vi "Verify threshold value by repeated iteration.vi"(4 "Cluster":T1={"Delta Matrix "=[[-1.0, 0.0, 0.0, 0.0, 0.0, 0.0, 0.0, 0.0, 0.0], [0.0, -1.0, 0.0, 0.0, 0.0, 0.0, 0.0, 0.0, 0.0], [0.0, 0.0, 0.0, 0.0, 0.0, 0.0, 0.0, 0.0, 0.0], [0.0, 0.0, 0.0, 0.0, 0.0, 0.0, 0.0, 0.0, 0.0], [10.0, 0.0, 0.0, 0.0, 0.0, 0.0, 0.0, 0.0, 0.0], [10.0, 0.0, 0.0, 0.0, 0.0, 0.0, 0.0, 0.0, 0.0], [0.0, 10.0, 0.0, 0.0, 0.0, 0.0, 0.0, 0.0, 0.0]], "Idx of Mod in Sp IDs "=[2, 8], "idx of OP "=0, "Init Sp State "=[], "Equations "=["kd*CI", "kd*GFP", "kd*LacI", "kd*TetR", "(ko__P1*ng__P1*Ko__P1*RNAP)/(1+Ko__P1*RNAP+(Kr__LacI_P1*LacI)^nc__LacI_P1)", "(ko__P2*ng__P2*Ko__P2*RNAP)/(1+Ko__P2*RNAP+(Kr__TetR_P2*TetR)^nc__TetR_P2)", "(ko__Promoter_GFP*ng__Promoter_GFP*Ko__Promoter_GFP*RNAP)/(1+Ko__Promoter_GFP*RNAP+(Kr__CI_Promoter_GFP*CI)^nc__CI_Promoter_GFP)"], "All Param Names "=[], "All Param Values "=[], "Sp Ids "=["CI", "GFP", "LacI", "P1", "P2", "P3", "P3_mRNA", "Promoter_GFP", "TetR"], "Start at "=0.0, "Pos Thresh "=10.0, "Runs "=0.0, "Init OP Conc "=0.0, "Comb "="", "Verification RT "=0.0, "CompID"=[], "CompSize"=[], "ModTimeSym"="", "Settling Time"=10}) -> (0 "T-Delay-SD":dbl format="%0.2f", 1 "OP Consistency":dbl, 2 "T-delay.av":i32)   [LabVIEW 2014]
doc: "This VI verifies the expected threshold value by iterating the model for the specified number of times. It also estimates the propogation delay (or input-output time delay). \n\nDesigned by HB\nhaba@dtu.dk"
uses:
  <vilib>/Analysis/Matrix/Datatypes/RealMatrix.ctl
  VerifyThreshInpCtrl.ctl
  ValSubsCtrl.ctl
  Trigger Status Bar.vi
  <vilib>/Analysis/Matrix/Numeric/Conversions/Matrix To Array - RM.vi
  <vilib>/gmath/NI_Gmath.lvlib
  <vilib>/Analysis/Matrix/NI_Matrix.lvlib
  <vilib>/Analysis/NI_AALBase.lvlib
panel:
  out "TIME IN MS":i32
  out "Time offset":i32=10
  out "T-Delay 2":dbl[](array[numeric])
  out "Zeros":dbl
  out "TD-Idxs":i32[](array[numeric])
  out "T-Delay":dbl[](array[numeric])
  out "Th-Var.av":dbl format="%0.2f"
  out "Th-SD.av":dbl format="%0.2f"
  out "Var":dbl[](array[numeric])
  out "SD":dbl[](array[numeric])
  out "ModTimeSym":string
  out "CompSize":string[](array[string])
  out "CompID":string[](array[string])
  out "Verification RT":dbl
  out "No. of inputs":i32
  out "Comb":string
  out "Init OP Conc":dbl
  out "Var Cnt":i32
  out "T-Delay Idx":i32
  out "Q":dbl
  out "O/p int Matrix":dbl[][](array[numeric]) format="%0.3f"
  out "Time int Matrix":dbl[][](array[numeric]) format="%0.3f"
  out "OP int data":dbl[](array[numeric])
  out "idx":i32
  out "T-Interval":dbl[](array[numeric])
  out "Q-Check":i32
  out "Time Matrix":dbl[][](array[numeric]) format="%0.3f"
  out "Time array":dbl[](array[numeric])
  in  "Print Interval":dbl=10.0
  out "OP Av":dbl[](array[numeric])
  out "Run":i32
  out "Init Sp State":i32[](array[numeric])
  out "Runs":dbl
  out "Log Data Nxt":dbl[](array[numeric])
  out "Log Data matrix 2":dbl[][](array[numeric]) format="%0.3f"
  out "OP Data":dbl[](array[numeric])
  out "O/p Matrix":dbl[][](array[numeric]) format="%0.3f"
  out "Pos Thresh":dbl=10.0
  out "Start at":dbl
  out "idx of OP":i32
  out "Mod data":dbl[](array[numeric])
  out "Sp Ids":string[](array[string])=["CI", "GFP", "LacI", "P1", "P2", "P3", "P3_mRNA", "Promoter_GFP", "TetR"]
  out "All Param Names":string[](array[string])
  out "All Param Values":string[](array[string])
  out "Nxt Sp State (N)":dbl[](array[numeric])
  out "Nxt Sp State (S)":string[](array[string])
  out "Idx of Mod in Sp IDs":i32[](array[numeric])=[2, 8]
  out "Nxt T":dbl
  out "Sum of Propensities for U":dbl
  out "Reac to execute":dbl[](array[numeric])
  out "Sum>a0*r2":bool
  out "Delta Matrix":T2=[[-1.0, 0.0, 0.0, 0.0, 0.0, 0.0, 0.0, 0.0, 0.0], [0.0, -1.0, 0.0, 0.0, 0.0, 0.0, 0.0, 0.0, 0.0], [0.0, 0.0, 0.0, 0.0, 0.0, 0.0, 0.0, 0.0, 0.0], [0.0, 0.0, 0.0, 0.0, 0.0, 0.0, 0.0, 0.0, 0.0], [10.0, 0.0, 0.0, 0.0, 0.0, 0.0, 0.0, 0.0, 0.0], [10.0, 0.0, 0.0, 0.0, 0.0, 0.0, 0.0, 0.0, 0.0], [0.0, 10.0, 0.0, 0.0, 0.0, 0.0, 0.0, 0.0, 0.0]]
  out "Reac IDx":i32
  out "a0*r2":dbl
  out "r1":dbl
  out "a0":dbl
  out "Propensities":dbl[](array[numeric])
  out "L_cnt":i32
  out "T":dbl[](array[numeric])
  out "tau":dbl
  out "r2":dbl
  out "Equations":string[](array[string])=["kd*CI", "kd*GFP", "kd*LacI", "kd*TetR", "(ko__P1*ng__P1*Ko__P1*RNAP)/(1+Ko__P1*RNAP+(Kr__LacI_P1*LacI)^nc__LacI_P1)", "(ko__P2*ng__P2*Ko__P2*RNAP)/(1+Ko__P2*RNAP+(Kr__TetR_P2*TetR)^nc__TetR_P2)", "(ko__Promoter_GFP*ng__Promoter_GFP*Ko__Promoter_GFP*RNAP)/(1+Ko__Promoter_GFP*RNAP+(Kr__CI_Promoter_GFP*CI)^nc__CI_Promoter_GFP)"]
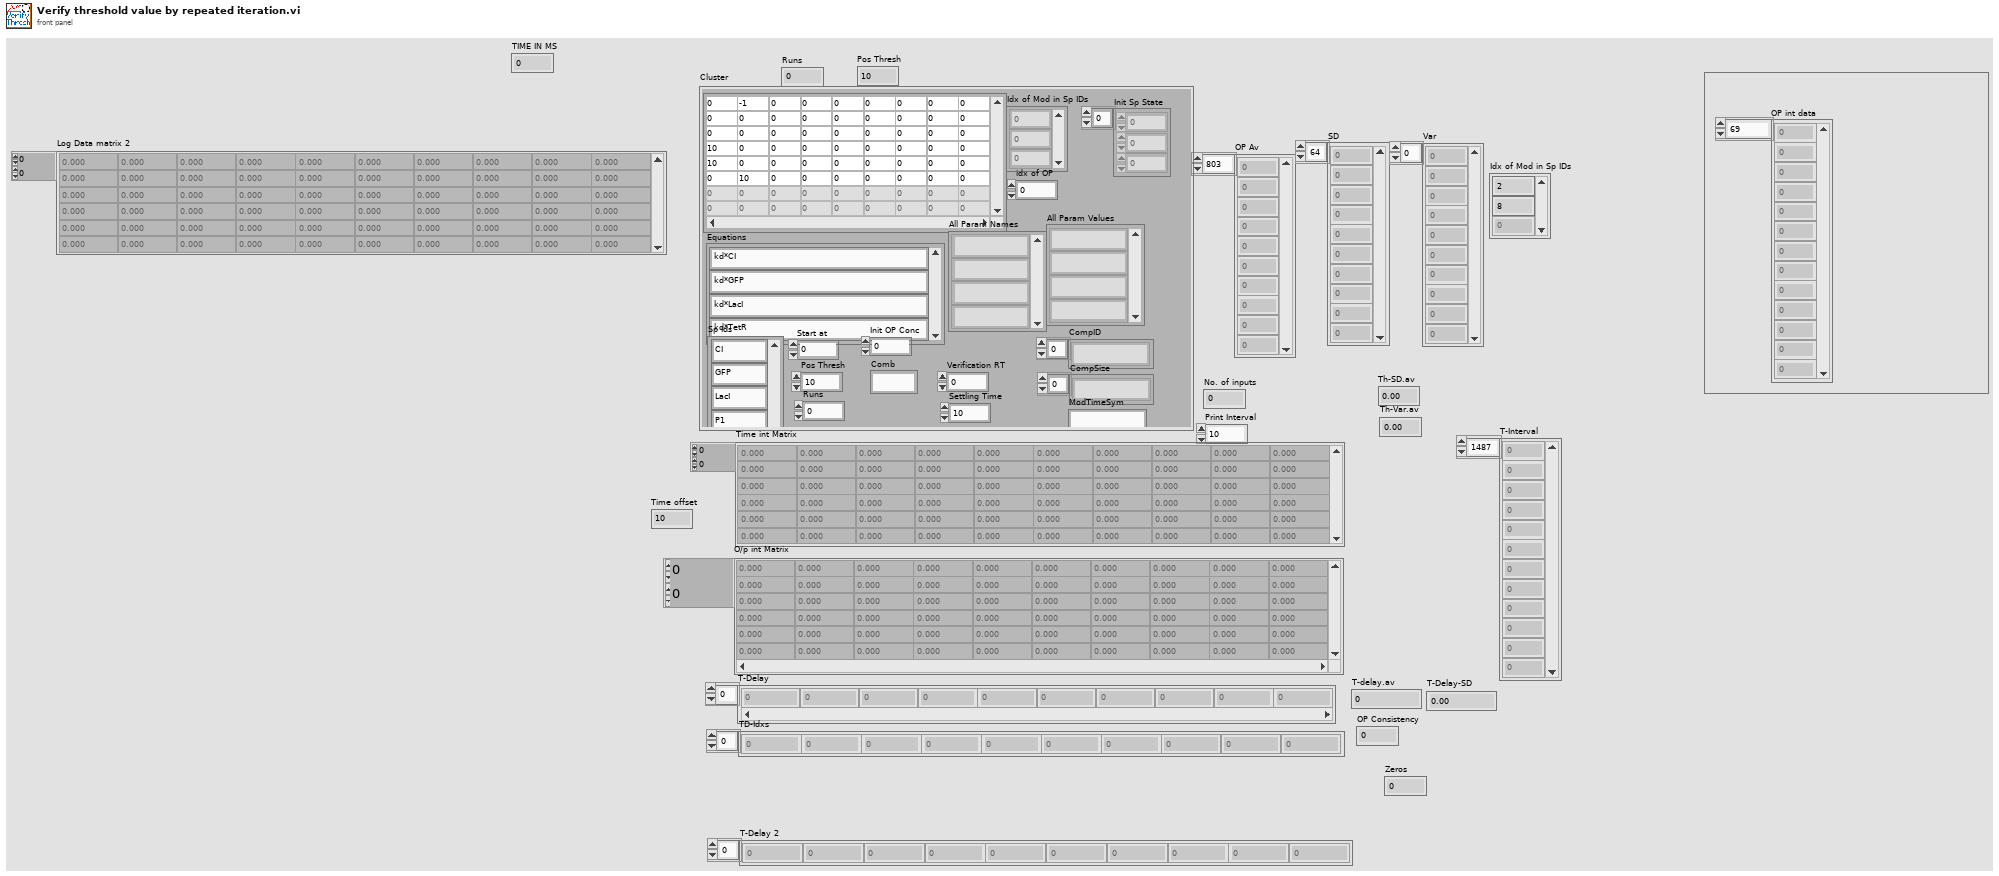
[diagram p1: front panel]
types:
  T1 = typedef "VerifyThreshInpCtrl.ctl" = cluster{"Delta Matrix ":T2, "Idx of Mod in Sp IDs ":i32[], "idx of OP ":i32, "Init Sp State ":i32[], "Equations ":string[], "All Param Names ":string[], "All Param Values ":string[], "Sp Ids ":string[], "Start at ":dbl, "Pos Thresh ":dbl, "Runs ":dbl, "Init OP Conc ":dbl, "Comb ":string, "Verification RT ":dbl, "CompID":string[], "CompSize":string[], "ModTimeSym":string, "Settling Time":i32}
  T2 = typedef "NI_Matrix.lvlib/RealMatrix.ctl" = dbl[][]
  T3 = typedef "ValSubsCtrl.ctl" = cluster{"All Param Names":string[], "All Param Values":string[], "Sp IDs":string[], "Sp States":string[], "Input Equations":string[], "CompID":string[], "CompSize":string[], "T-Sym":string, "T":dbl}
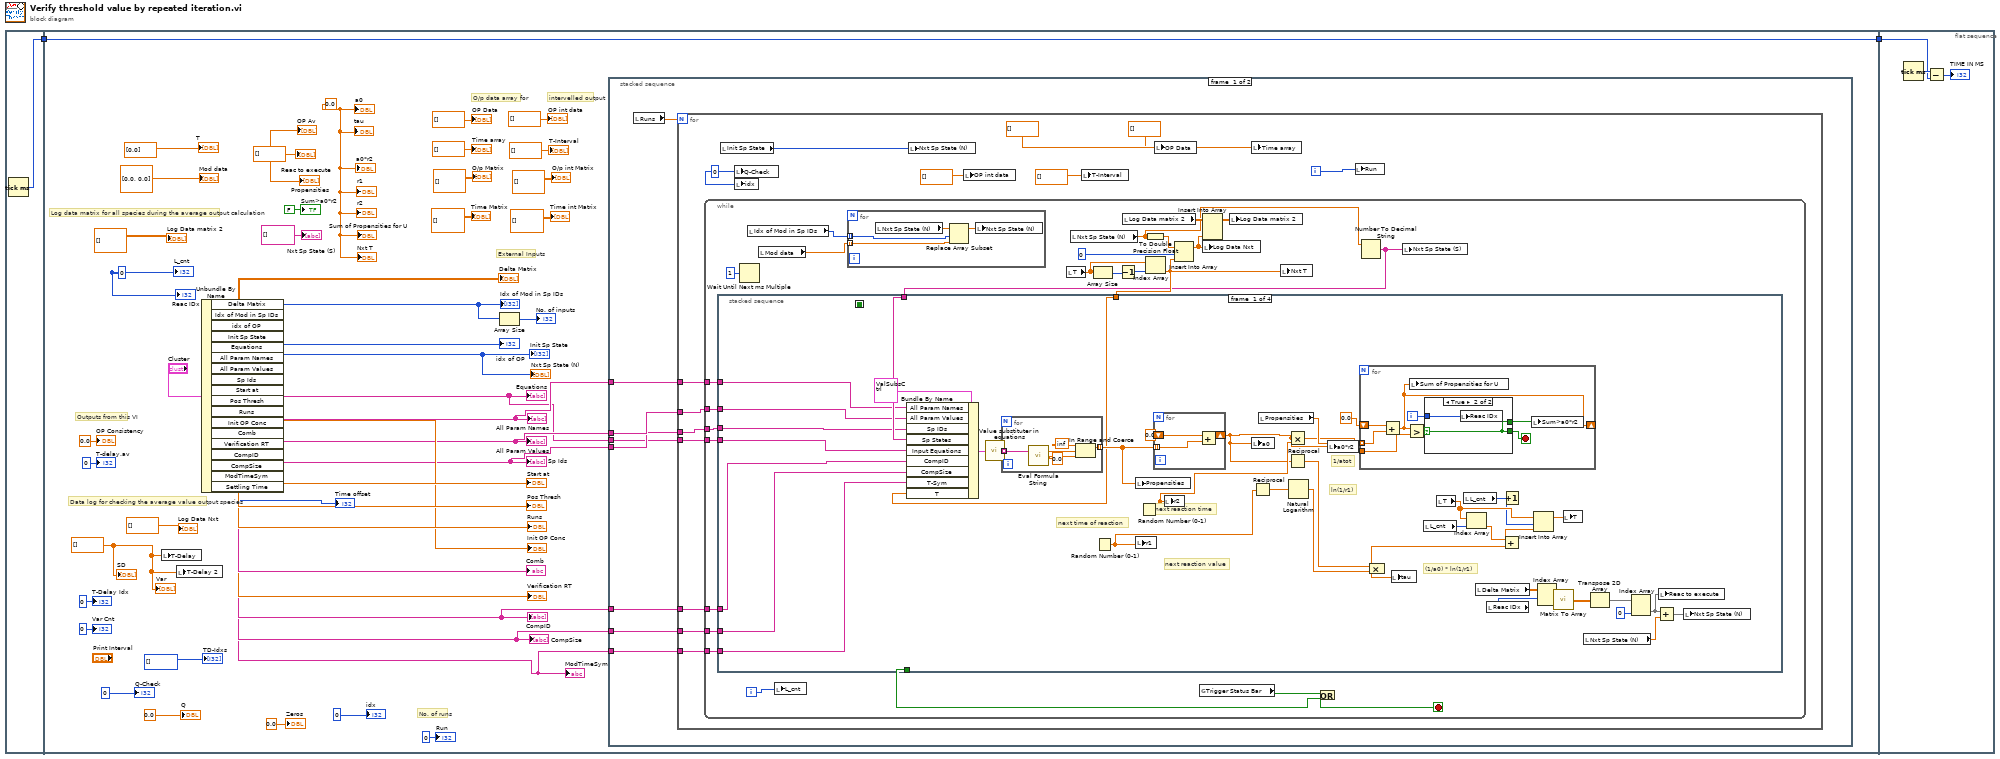
[diagram p0: block diagram]
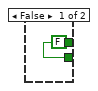
[diagram p2: hidden frame]
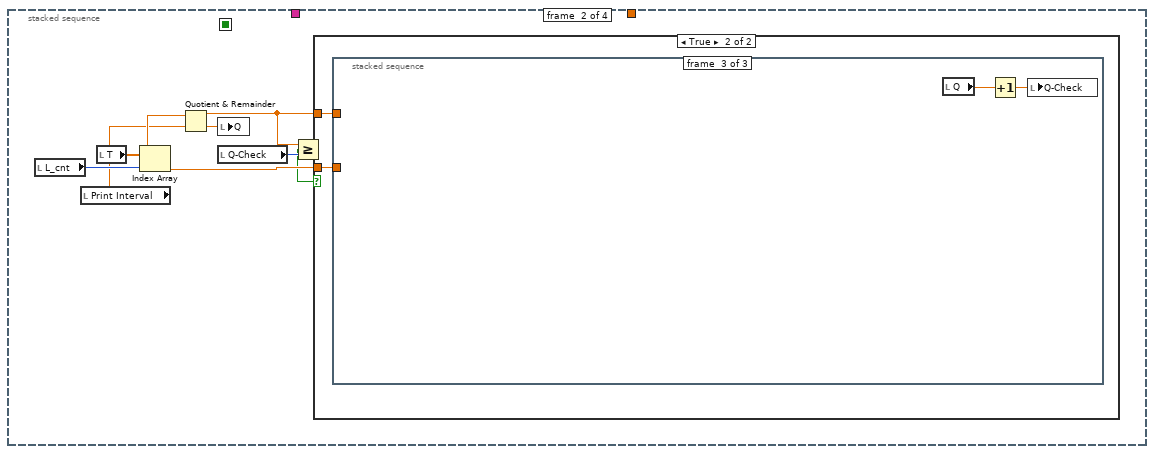
[diagram p3: hidden frame]
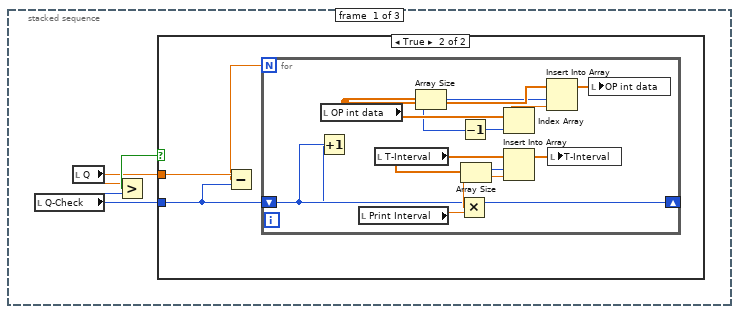
[diagram p5: hidden frame]
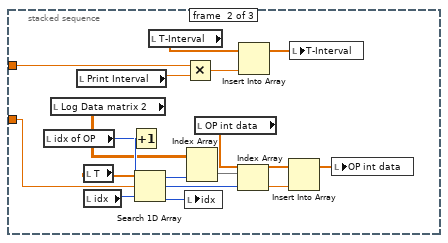
[diagram p7: hidden frame]
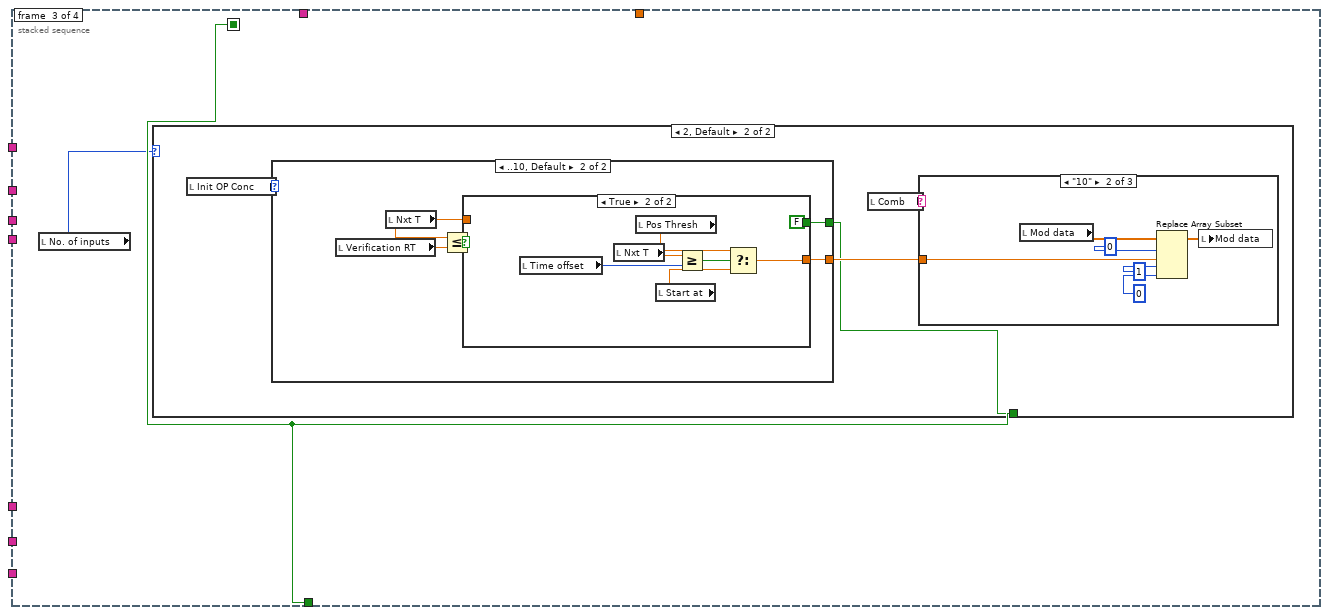
[diagram p8: hidden frame]
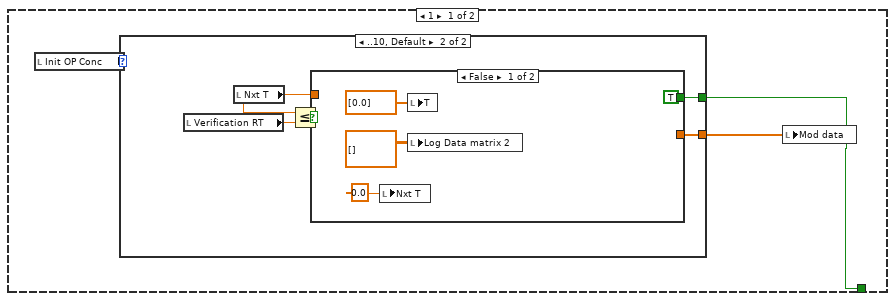
[diagram p9: hidden frame]
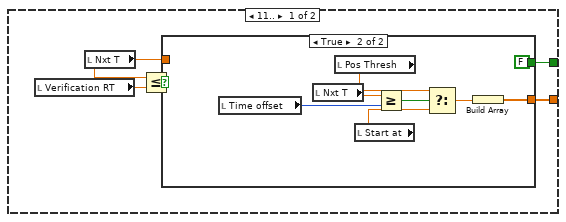
[diagram p10: hidden frame]
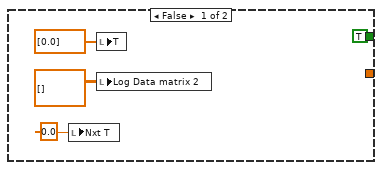
[diagram p11: hidden frame]
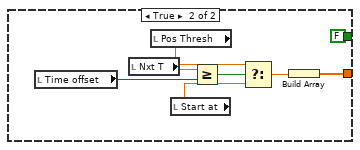
[diagram p12: hidden frame]
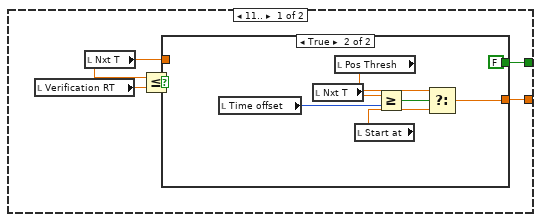
[diagram p13: hidden frame]
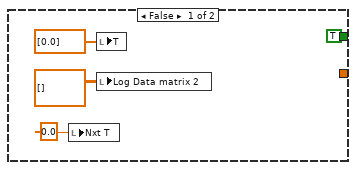
[diagram p14: hidden frame]
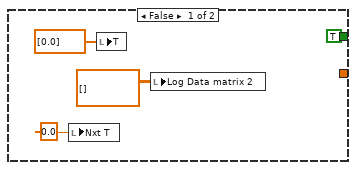
[diagram p15: hidden frame]
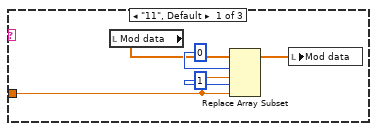
[diagram p16: hidden frame]
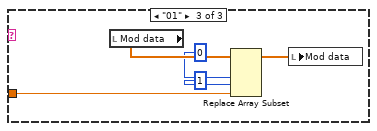
[diagram p17: hidden frame]
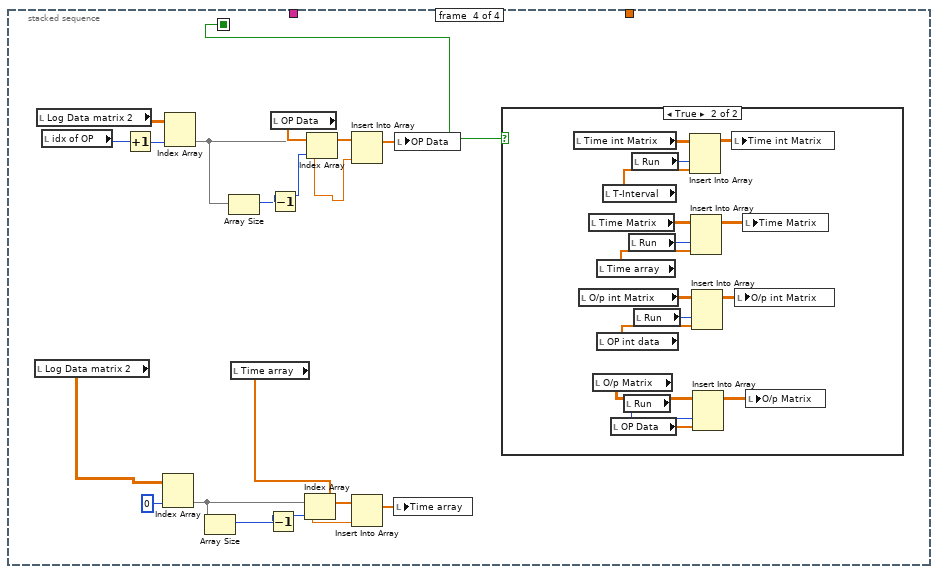
[diagram p18: hidden frame]
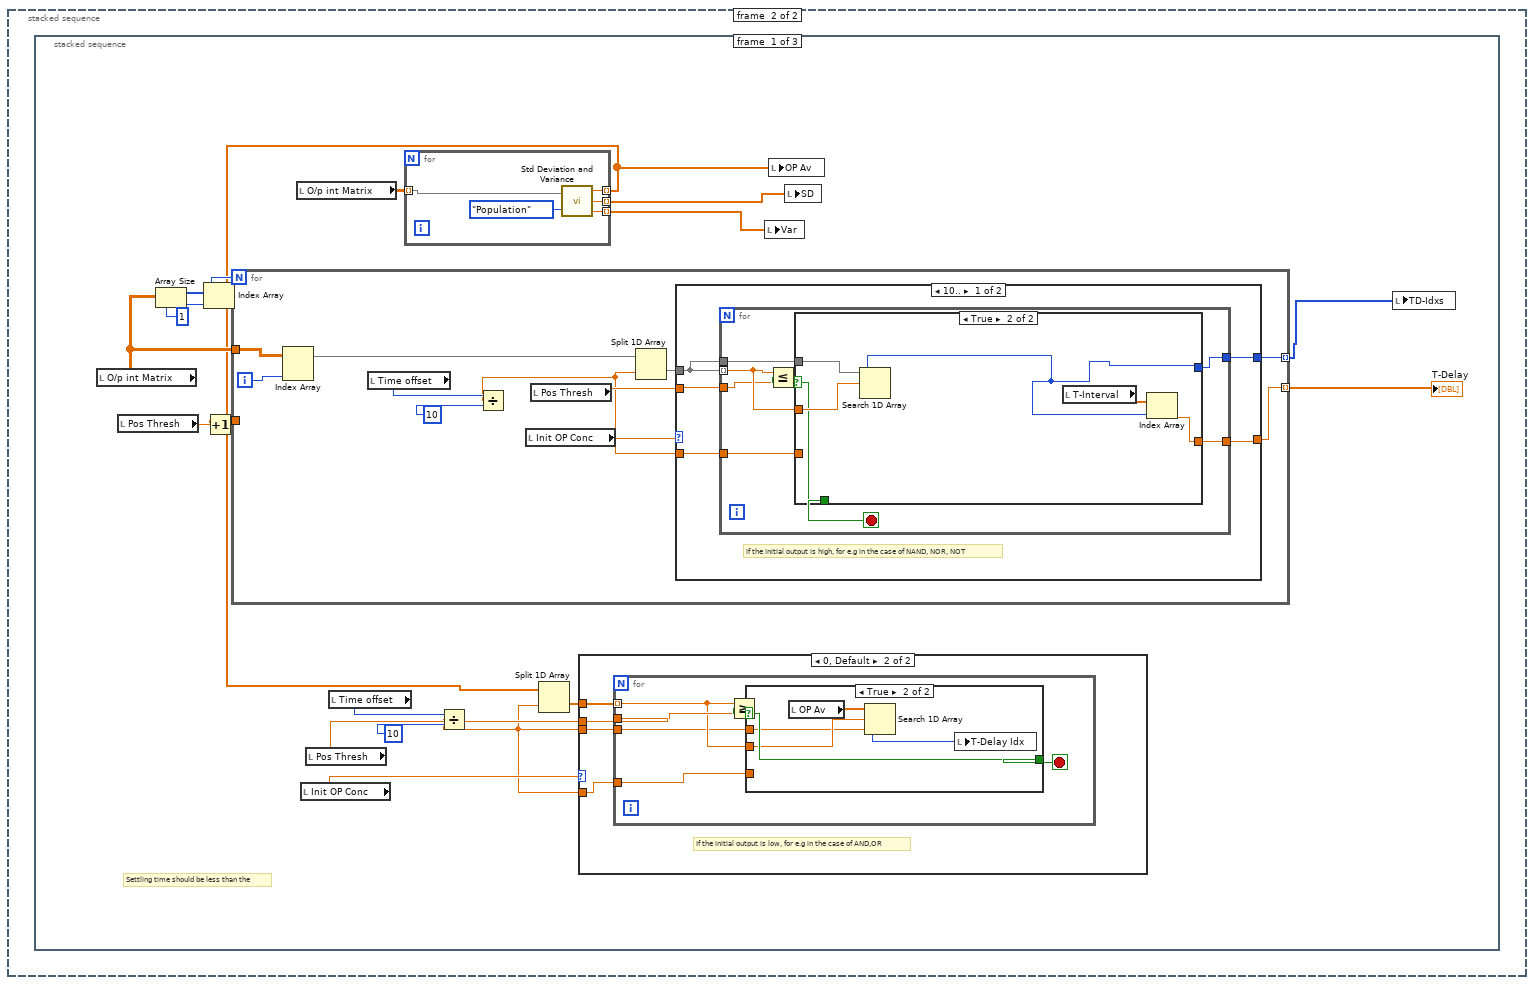
[diagram p20: hidden frame]
diagram:
  n1 = flat-sequence {
    tunnel: [w3] -> w1
    tunnel: [w11] -> w2
    tunnel: w1 -> [w11]
    tunnel: w2 -> [w514]
    frame #0 {
      n2 = Tick Count (ms)() -> (millisecond timer value=w3:u32)
    }
    frame #1 {
      w13 = dbl[] [] ("Var")
      w43 = 0 ("L_cnt")
      w41 = dbl[] [] ("Reac to execute")
      w47 = 0.0 ("a0")
      # "Outputs from this VI"
      # "intervelled output"
      # "No. of runs"
      # "External Inputs"
      # "O/p data array for"
      # "Log data matrix for all species during the average output calculation"
      # "Data log for checking the average value output species"
      n3 = local write "T-Delay"(w13) -> ()
      n4 = local write "T-Delay 2"(w13) -> ()
      n5 = Unbundle By Name("Cluster") -> ("Delta Matrix"=→"Delta Matrix":T2, "Idx of Mod in Sp IDs"=w24:i32[], "idx of OP"=→"idx of OP":i32, "Init Sp State"=→"Nxt Sp State (N)" →"Init Sp State":i32[], "Equations"=w7:string[], "All Param Names"=w10:string[], "All Param Values"=w9:string[], "Sp Ids"=w8:string[], "Start at"=→"Start at":dbl, "Pos Thresh"=→"Pos Thresh":dbl, "Runs"=→"Runs":dbl, "Init OP Conc"=→"Init OP Conc":dbl, "Comb"=→"Comb":string, "Verification RT"=→"Verification RT":dbl, "CompID"=w6:string[], "CompSize"=w5:string[], "ModTimeSym"=w4:string, "Settling Time"=→"Time offset":i32)
      "Equations" <- w7
      "Idx of Mod in Sp IDs" <- w24
      "All Param Values" <- w9
      "All Param Names" <- w10
      "Sp Ids" <- w8
      "CompID" <- w6
      "CompSize" <- w5
      "ModTimeSym" <- w4
      n6 = Array Size(array=w24) -> (size(s)=→"No. of inputs":i32)
      n7 = stacked-sequence {
        tunnel: w10 -> [w59 _]
        tunnel: w9 -> [w58 _]
        tunnel: w8 -> [w57 _]
        tunnel: w7 -> [w56 _]
        tunnel: w6 -> [w55 _]
        tunnel: w5 -> [w54 _]
        tunnel: w4 -> [w53 _]
        frame #0 {
          n8 = local read "Runs"() -> (w60:dbl)
          n9 = for {
            N: w60 -> [_]
            tunnel: w59 -> [w67]
            tunnel: w58 -> [w66]
            tunnel: w57 -> [w65]
            tunnel: w56 -> [w64]
            tunnel: w55 -> [w63]
            tunnel: w54 -> [w62]
            tunnel: w53 -> [w61]
            i -> [w73]
            w68 = 0 ("Q-Check")
            n10 = while {
              tunnel: w67 -> [w81]
              tunnel: w66 -> [w80]
              tunnel: w65 -> [w79]
              tunnel: w64 -> [w78]
              tunnel: w63 -> [w77]
              tunnel: w62 -> [w76]
              tunnel: w61 -> [w75]
              i -> [w99]
              stop <- w95 stop-if-true
              n11 = Wait Until Next ms Multiple(millisecond multiple=u32 1) -> ()  [unwired: 1 out]
              n12 = local read "Idx of Mod in Sp IDs"() -> (w93:i32[])
              n13 = local read "Mod data"() -> (w94:dbl[])
              n14 = local write "L_cnt"(w99) -> ()
              n15 = for {
                tunnel: w93 -> [w102] mode=indexing
                tunnel: w94 -> [w100] mode=indexing
                n16 = local read "Nxt Sp State (N)"() -> (w103:dbl[])
                n17 = Replace Array Subset(array=w103, new element=w100, index=w102) -> (w101:dbl[])
                n18 = local write "Nxt Sp State (N)"(w101) -> ()
              }
              n19 = local read "T"() -> (w92:dbl[])
              n20 = local read "Nxt Sp State (N)"() -> (w84:dbl[])
              n21 = Array Size(array=w92) -> (size(s)=w91:i32)
              n22 = Decrement(x=w91) -> (x-1=w90:i32)
              n23 = local read "Log Data matrix 2"() -> (w87:dbl[][])
              n24 = To Double Precision Float(number=w84) -> (double precision float=w88:dbl[])
              n25 = Index Array(array=w92, index=w90) -> (element=w83:dbl)
              n26 = Insert Into Array(array=w88, index=0, new element=w83) -> (w85:dbl[])
              n27 = global read "Trigger Status Bar.vi" "Trigger Status Bar"() -> (w96:bool)
              n28 = Insert Into Array(array=w87, new element=w85) -> (w86:dbl[][])  [unwired: 2 in]
              n29 = local write "Log Data Nxt"(w85) -> ()
              n30 = local write "Log Data matrix 2"(w86) -> ()
              n31 = local write "Nxt T"(w83) -> ()
              n32 = Number To Decimal String(number=w84) -> (decimal integer string=w82:string[])  [unwired: 1 in]
              n33 = stacked-sequence {
                seq-local: [_ _ w209 _] -> [_ _ _ w313]
                tunnel: [_ _ w209 _] -> w97
                tunnel: w83 -> [w112 _ _ _]
                tunnel: w82 -> [w111 _ _ _]
                tunnel: w81 -> [w110 _ _ _]
                tunnel: w80 -> [w109 _ _ _]
                tunnel: w79 -> [w108 _ _ _]
                tunnel: w78 -> [w107 _ _ _]
                tunnel: w77 -> [w106 _ _ _]
                tunnel: w76 -> [w105 _ _ _]
                tunnel: w75 -> [w104 _ _ _]
                frame #0 {
                  # "next time of reaction"
                  # "next reaction value"
                  # "(1/a0) * ln(1/r1)"
                  # "1/atot"
                  # "ln(1/r1)"
                  # "next reaction time"
                  n34 = Bundle By Name(cluster=T3 {"All Param Names"=["k1"], "All Param Values"=["1.5"], "Sp IDs"=["S1", "S2", "S3"], "Sp States"=["0.000000", "0.000000", "0.000000"], "Input Equations"=["C*k1*S1", "1.5*exp(time)^(-1)"], "CompID"=["C"], "CompSize"=["3.0"], "T-Sym"="time", "T"=0.0} ("Cluster"), "All Param Names"=w110, "All Param Values"=w109, "Sp IDs"=w108, "Sp States"=w111, "Input Equations"=w107, "CompID"=w106, "CompSize"=w105, "T-Sym"=w104, "T"=w112) -> (w140:T3)
                  n35 = call "Value substituter in equations.vi"("Cluster"=w140) -> ("Output Equations"=w143:string[])
                  n36 = for {
                    tunnel: w143 -> [w162] mode=indexing
                    tunnel: [w158] -> w142 mode=indexing
                    n37 = call <vilib>:"Eval Formula String.vi"("formula"=w162) -> ("y value"=w159:dbl)  [unwired: 1 in, 1 out]
                    n38 = In Range and Coerce(upper limit=inf, x=w159, lower limit=0.0) -> (coerced(x)=w158:dbl)  [unwired: 1 out]
                  }
                  n39 = Random Number (0-1)() -> (number: 0 to 1=w136:dbl)
                  n40 = local write "Propensities"(w142) -> ()
                  n41 = local write "r1"(w136) -> ()
                  n42 = Random Number (0-1)() -> (number: 0 to 1=w137:dbl)
                  n43 = for {
                    tunnel: w142 -> [w157] mode=indexing
                    shift-right: [w156] -> w126
                    shift-left: 0.0 -> [w155]
                    n44 = Add(x=w155, y=w157) -> (x+y=w156:dbl)
                  }
                  n45 = local write "r2"(w137) -> ()
                  n46 = local write "a0"(w126) -> ()
                  n47 = Reciprocal(x=w136) -> (1/x=w127:dbl)
                  n48 = local read "Propensities"() -> (w124:dbl[])
                  n49 = Multiply(x=w126, y=w137) -> (x*y=w123:dbl)
                  n50 = Reciprocal(x=w126) -> (1/x=w128:dbl)
                  n51 = Natural Logarithm(1:w127) -> (0:w129:dbl)
                  n52 = local write "a0*r2"(w123) -> ()
                  n53 = for {
                    tunnel: w124 -> [w148] mode=indexing
                    shift-right: [w147] -> _
                    shift-left: 0.0 -> [w151]
                    tunnel: w123 -> [w144]
                    i -> [w145]
                    stop <- w149 stop-if-true
                    n54 = Add(x=w151, y=w148) -> (x+y=w147:dbl)
                    n55 = Greater?(x=w147, y=w144) -> (0:w150:bool)
                    n56 = local write "Sum of Propensities for U"(w147) -> ()
                    n57 = case shown="True" w150 {
                      selector: w150 -> [_ w154]
                      tunnel: [w152 w154] -> w149
                      tunnel: [w152 w154] -> w146
                      tunnel: w145 -> [_ w153]
                      frame False {
                        w152 = FALSE
                      }
                      frame True {
                        n58 = local write "Reac IDx"(w153) -> ()
                      }
                    }
                    n59 = local write "Sum>a0*r2"(w146) -> ()
                  }
                  n60 = Compound Arithmetic op=MULTIPLY(w128, w129) -> (w122:dbl)
                  n61 = local write "tau"(w122) -> ()
                  n62 = local read "L_cnt"() -> (w132:i32)
                  n63 = local read "T"() -> (w138:dbl[])
                  n64 = local read "L_cnt"() -> (w134:i32)
                  n65 = Index Array(array=w138, index=w132) -> (element=w131:dbl)
                  n66 = local read "Delta Matrix"() -> (w113:T2)
                  n67 = local read "Reac IDx"() -> (w114:i32)
                  n68 = Add(x=w131, y=w122) -> (x+y=w133:dbl)
                  n69 = Increment(x=w134) -> (x+1=w130:i32)
                  n70 = Insert Into Array(array=w138, index=w130, new element=w133) -> (w135:dbl[])
                  n71 = Index Array(array=w113, index (row)=w114) -> (element=w115:T2)  [unwired: 1 in]
                  n72 = call-poly <vilib>:"Matrix To Array.vi"("Real Matrix"=w115) -> ("Real 2D Array"=w116:dbl[][])
                  n73 = local write "T"(w135) -> ()
                  n74 = local read "Nxt Sp State (N)"() -> (w119:dbl[])
                  n75 = Transpose 2D Array(2D array=w116) -> (transposed array=w117:dbl[][])
                  n76 = Index Array(array=w117, index (col)=0 ("disabled index (col)")) -> (element=w121:dbl[])  [unwired: 1 in]
                  n77 = Add(x=w121, y=w119) -> (x+y=w120:dbl[])
                  n78 = local write "Reac to execute"(w121) -> ()
                  n79 = local write "Nxt Sp State (N)"(w120) -> ()
                }
                frame #1 {
                  n80 = local read "L_cnt"() -> (w168:i32)
                  n81 = local read "Print Interval"() -> (w166:dbl)
                  n82 = local read "T"() -> (w167:dbl[])
                  n83 = Index Array(array=w167, index=w168) -> (element=w169:dbl)
                  n84 = Quotient & Remainder(x=w169, y=w166) -> (floor(x/y)=w163:dbl)  [unwired: 1 out]
                  n85 = local write "Q"(w163) -> ()
                  n86 = local read "Q-Check"() -> (w165:i32)
                  n87 = Greater Or Equal?(x=w163, y=w165) -> (x >= y?=w164:bool)
                  n88 = case shown="True" w164 {
                    tunnel: w169 -> [_ w171]
                    tunnel: w163 -> [_ w170]
                    frame False {
                    }
                    frame True {
                      n89 = stacked-sequence {
                        tunnel: w171 -> [_ w204 _]
                        tunnel: w170 -> [_ w190 _]
                        frame #0 {
                          n90 = local read "Q-Check"() -> (w172:i32)
                          n91 = local read "Q"() -> (w173:dbl)
                          n92 = Greater?(x=w173, y=w172) -> (0:w174:bool)
                          n93 = case shown="True" w174 {
                            tunnel: w173 -> [_ w177]
                            tunnel: w172 -> [_ w175]
                            frame False {
                            }
                            frame True {
                              n94 = Subtract(x=w177, y=w175) -> (x-y=w176:dbl)
                              n95 = for {
                                N: w176 -> [_]
                                shift-right: [w184] -> _
                                shift-left: w175 -> [w185]
                                n96 = Increment(x=w185) -> (x+1=w184:i32)
                                n97 = local read "OP int data"() -> (w182:dbl[])
                                n98 = local read "Print Interval"() -> (w189:dbl)
                                n99 = local read "T-Interval"() -> (w186:dbl[])
                                n100 = Array Size(array=w182) -> (size(s)=w178:i32)
                                n101 = Multiply(x=w185, y=w189) -> (x*y=w187:dbl)
                                n102 = Decrement(x=w178) -> (x-1=w181:i32)
                                n103 = Array Size(array=w186) -> (size(s)=w179:i32)
                                n104 = Index Array(array=w182, index=w181) -> (element=w180:dbl)
                                n105 = Insert Into Array(array=w186, index=w179, new element=w187) -> (w188:dbl[])
                                n106 = Insert Into Array(array=w182, index=w178, new element=w180) -> (w183:dbl[])
                                n107 = local write "T-Interval"(w188) -> ()
                                n108 = local write "OP int data"(w183) -> ()
                              }
                            }
                          }
                        }
                        frame #1 {
                          n109 = local read "idx of OP"() -> (w201:i32)
                          n110 = local read "Log Data matrix 2"() -> (w200:dbl[][])
                          n111 = local read "Print Interval"() -> (w191:dbl)
                          n112 = local read "T"() -> (w205:dbl[])
                          n113 = local read "idx"() -> (w203:i32)
                          n114 = Increment(x=w201) -> (x+1=w202:i32)
                          n115 = Search 1D Array(1D array=w205, element=w204, start index (0)=w203) -> (index of element=w198:i32)
                          n116 = local read "T-Interval"() -> (w193:dbl[])
                          n117 = Multiply(x=w190, y=w191) -> (x*y=w192:dbl)
                          n118 = local write "idx"(w198) -> ()
                          n119 = Index Array(array=w200, index (col)=w202) -> (element=w199:dbl[])  [unwired: 1 in]
                          n120 = local read "OP int data"() -> (w197:dbl[])
                          n121 = Index Array(array=w199, index=w198) -> (element=w195:dbl)
                          n122 = Insert Into Array(array=w193, new element=w192) -> (w194:dbl[])  [unwired: 1 in]
                          n123 = Insert Into Array(array=w197, new element=w195) -> (w196:dbl[])  [unwired: 1 in]
                          n124 = local write "T-Interval"(w194) -> ()
                          n125 = local write "OP int data"(w196) -> ()
                        }
                        frame #2 {
                          n126 = local read "Q"() -> (w207:dbl)
                          n127 = Increment(x=w207) -> (x+1=w206:dbl)
                          n128 = local write "Q-Check"(w206) -> ()
                        }
                      }
                    }
                  }
                }
                frame #2 {
                  n129 = local read "No. of inputs"() -> (w208:i32)
                  n130 = case shown="2, Default" w208 {
                    tunnel: [w211 w249] -> w209
                    frame 1 {
                      n131 = local read "Init OP Conc"() -> (w212:dbl)
                      n132 = case shown="..10, Default" w212 {
                        tunnel: [w217 w230] -> w210
                        tunnel: [w216 w234] -> w211
                        frame 11.. {
                          n133 = local read "Verification RT"() -> (w213:dbl)
                          n134 = local read "Nxt T"() -> (w214:dbl)
                          n135 = Less Or Equal?(x=w214, y=w213) -> (x <= y?=w215:bool)
                          n136 = case shown="True" w215 {
                            tunnel: [_ w229] -> w217
                            tunnel: [TRUE FALSE] -> w216
                            tunnel: w214 -> [_ _]
                            frame False {
                              n137 = local write "Nxt T"(0.0 ("Nxt T")) -> ()
                              n138 = local write "T"(dbl[] [0.0] ("T")) -> ()
                              n139 = local write "Log Data matrix 2"(dbl[][] [] ("Log Data matrix")) -> ()
                            }
                            frame True {
                              n140 = local read "Time offset"() -> (w222:i32)
                              n141 = local read "Nxt T"() -> (w225:dbl)
                              n142 = local read "Pos Thresh"() -> (w226:dbl)
                              n143 = local read "Start at"() -> (w227:dbl)
                              n144 = Greater Or Equal?(x=w225, y=w222) -> (x >= y?=w224:bool)
                              n145 = Select(t=w226, s=w224, f=w227) -> (s? t:f=w223:dbl)
                              n146 = Build Array(w223) -> (w229:dbl[])
                            }
                          }
                        }
                        frame ..10, Default {
                          n147 = local read "Verification RT"() -> (w231:dbl)
                          n148 = local read "Nxt T"() -> (w232:dbl)
                          n149 = Less Or Equal?(x=w232, y=w231) -> (x <= y?=w233:bool)
                          n150 = case shown="False" w233 {
                            tunnel: [_ w246] -> w230
                            tunnel: [TRUE FALSE] -> w234
                            tunnel: w232 -> [_ _]
                            frame False {
                              n151 = local write "Nxt T"(0.0 ("Nxt T")) -> ()
                              n152 = local write "T"(dbl[] [0.0] ("T")) -> ()
                              n153 = local write "Log Data matrix 2"(dbl[][] [] ("Log Data matrix")) -> ()
                            }
                            frame True {
                              n154 = local read "Time offset"() -> (w239:i32)
                              n155 = local read "Nxt T"() -> (w242:dbl)
                              n156 = local read "Pos Thresh"() -> (w243:dbl)
                              n157 = local read "Start at"() -> (w244:dbl)
                              n158 = Greater Or Equal?(x=w242, y=w239) -> (x >= y?=w241:bool)
                              n159 = Select(t=w243, s=w241, f=w244) -> (s? t:f=w240:dbl)
                              n160 = Build Array(w240) -> (w246:dbl[])
                            }
                          }
                        }
                      }
                      n161 = local write "Mod data"(w210) -> ()
                    }
                    frame 2, Default {
                      n162 = local read "Init OP Conc"() -> (w247:dbl)
                      n163 = case shown="..10, Default" w247 {
                        tunnel: [w255 w271] -> w250
                        tunnel: [w254 w270] -> w249
                        frame 11.. {
                          n164 = local read "Verification RT"() -> (w251:dbl)
                          n165 = local read "Nxt T"() -> (w252:dbl)
                          n166 = Less Or Equal?(x=w252, y=w251) -> (x <= y?=w253:bool)
                          n167 = case shown="True" w253 {
                            tunnel: [_ w261] -> w255
                            tunnel: [TRUE FALSE] -> w254
                            tunnel: w252 -> [_ _]
                            frame False {
                              n168 = local write "Nxt T"(0.0 ("Nxt T")) -> ()
                              n169 = local write "T"(dbl[] [0.0] ("T")) -> ()
                              n170 = local write "Log Data matrix 2"(dbl[][] [] ("Log Data matrix")) -> ()
                            }
                            frame True {
                              n171 = local read "Time offset"() -> (w260:i32)
                              n172 = local read "Nxt T"() -> (w263:dbl)
                              n173 = local read "Pos Thresh"() -> (w264:dbl)
                              n174 = local read "Start at"() -> (w265:dbl)
                              n175 = Greater Or Equal?(x=w263, y=w260) -> (x >= y?=w262:bool)
                              n176 = Select(t=w264, s=w262, f=w265) -> (s? t:f=w261:dbl)
                            }
                          }
                        }
                        frame ..10, Default {
                          n177 = local read "Verification RT"() -> (w267:dbl)
                          n178 = local read "Nxt T"() -> (w268:dbl)
                          n179 = Less Or Equal?(x=w268, y=w267) -> (x <= y?=w269:bool)
                          n180 = case shown="True" w269 {
                            tunnel: [_ w277] -> w271
                            tunnel: [TRUE FALSE] -> w270
                            tunnel: w268 -> [_ _]
                            frame False {
                              n181 = local write "Nxt T"(0.0 ("Nxt T")) -> ()
                              n182 = local write "T"(dbl[] [0.0] ("T")) -> ()
                              n183 = local write "Log Data matrix 2"(dbl[][] [] ("Log Data matrix")) -> ()
                            }
                            frame True {
                              n184 = local read "Time offset"() -> (w276:i32)
                              n185 = local read "Nxt T"() -> (w279:dbl)
                              n186 = local read "Pos Thresh"() -> (w280:dbl)
                              n187 = local read "Start at"() -> (w281:dbl)
                              n188 = Greater Or Equal?(x=w279, y=w276) -> (x >= y?=w278:bool)
                              n189 = Select(t=w280, s=w278, f=w281) -> (s? t:f=w277:dbl)
                            }
                          }
                        }
                      }
                      n190 = local read "Comb"() -> (w248:string)
                      n191 = case shown="\"10\"" w248 {
                        tunnel: w250 -> [w283 w289 w295]
                        frame "11", Default {
                          n192 = local read "Mod data"() -> (w285:dbl[])
                          n193 = Replace Array Subset(array=w285, new element #1=w283, index #1=0 ("index"), new element #2=w283, index #2=1 ("index")) -> (w284:dbl[])
                          n194 = local write "Mod data"(w284) -> ()
                        }
                        frame "10" {
                          n195 = local read "Mod data"() -> (w291:dbl[])
                          n196 = Replace Array Subset(array=w291, new element #1=w289, index #1=0 ("index"), new element #2=0 ("index"), index #2=1 ("index")) -> (w290:dbl[])
                          n197 = local write "Mod data"(w290) -> ()
                        }
                        frame "01" {
                          n198 = local read "Mod data"() -> (w297:dbl[])
                          n199 = Replace Array Subset(array=w297, new element #1=0 ("index"), new element #2=w295, index #2=1 ("index")) -> (w296:dbl[])  [unwired: 1 in]
                          n200 = local write "Mod data"(w296) -> ()
                        }
                      }
                    }
                  }
                }
                frame #3 {
                  n201 = local read "Log Data matrix 2"() -> (w300:dbl[][])
                  n202 = local read "Log Data matrix 2"() -> (w316:dbl[][])
                  n203 = local read "idx of OP"() -> (w315:i32)
                  n204 = Increment(x=w315) -> (x+1=w314:i32)
                  n205 = Index Array(array=w300, index (col)=0 ("disabled index (col)")) -> (element=w304:dbl[])  [unwired: 1 in]
                  n206 = Index Array(array=w316, index (col)=w314) -> (element=w309:dbl[])  [unwired: 1 in]
                  n207 = Array Size(array=w304) -> (size(s)=w305:i32)
                  n208 = Array Size(array=w309) -> (size(s)=w308:i32)
                  n209 = local read "Time array"() -> (w301:dbl[])
                  n210 = Decrement(x=w305) -> (x-1=w303:i32)
                  n211 = Decrement(x=w308) -> (x-1=w310:i32)
                  n212 = local read "OP Data"() -> (w312:dbl[])
                  n213 = Index Array(array=w304, index=w303) -> (element=w306:dbl)
                  n214 = Index Array(array=w309, index=w310) -> (element=w307:dbl)
                  n215 = Insert Into Array(array=w312, new element=w307) -> (w311:dbl[])  [unwired: 1 in]
                  n216 = Insert Into Array(array=w301, new element=w306) -> (w302:dbl[])  [unwired: 1 in]
                  n217 = local write "Time array"(w302) -> ()
                  n218 = local write "OP Data"(w311) -> ()
                  n219 = case shown="True" w313 {
                    frame False {
                    }
                    frame True {
                      n220 = local read "Time int Matrix"() -> (w324:dbl[][])
                      n221 = local read "O/p int Matrix"() -> (w317:dbl[][])
                      n222 = local read "Time Matrix"() -> (w325:dbl[][])
                      n223 = local read "O/p Matrix"() -> (w332:dbl[][])
                      n224 = local read "Time array"() -> (w328:dbl[])
                      n225 = local read "OP int data"() -> (w320:dbl[])
                      n226 = local read "T-Interval"() -> (w321:dbl[])
                      n227 = local read "OP Data"() -> (w329:dbl[])
                      n228 = local read "Run"() -> (w330:i32)
                      n229 = local read "Run"() -> (w327:i32)
                      n230 = local read "Run"() -> (w322:i32)
                      n231 = local read "Run"() -> (w319:i32)
                      n232 = Insert Into Array(array=w324, index (col)=w322, new element=w321) -> (w323:dbl[][])  [unwired: 1 in]
                      n233 = Insert Into Array(array=w325, index (col)=w327, new element=w328) -> (w326:dbl[][])  [unwired: 1 in]
                      n234 = Insert Into Array(array=w317, index (col)=w319, new element=w320) -> (w318:dbl[][])  [unwired: 1 in]
                      n235 = Insert Into Array(array=w332, index (col)=w330, new element=w329) -> (w331:dbl[][])  [unwired: 1 in]
                      n236 = local write "Time int Matrix"(w323) -> ()
                      n237 = local write "O/p int Matrix"(w318) -> ()
                      n238 = local write "Time Matrix"(w326) -> ()
                      n239 = local write "O/p Matrix"(w331) -> ()
                    }
                  }
                }
              }
              n240 = Or(x=w96, y=w97) -> (x .or. y?=w95:bool)
              n241 = local write "Nxt Sp State (S)"(w82) -> ()
            }
            n242 = local read "Init Sp State"() -> (w74:i32[])
            n243 = local write "Q-Check"(w68) -> ()
            n244 = local write "idx"(w68) -> ()
            n245 = local write "Nxt Sp State (N)"(w74) -> ()
            n246 = local write "OP int data"(dbl[] [] ("OP Data 2")) -> ()
            n247 = local write "T-Interval"(dbl[] [] ("OP Data 2")) -> ()
            n248 = local write "OP Data"(dbl[] [] ("OP Data 2")) -> ()
            n249 = local write "Time array"(dbl[] [] ("OP Data 2")) -> ()
            n250 = local write "Run"(w73) -> ()
          }
        }
        frame #1 {
          n251 = stacked-sequence {
            frame #0 {
              # "Settling time should be less than the"
              n252 = local read "O/p int Matrix"() -> (w343:dbl[][])
              n253 = local read "Pos Thresh"() -> (w338:dbl)
              n254 = Array Size(array=w343) -> (size(s)=w342:i32[])
              n255 = Index Array(array=w342, index=1) -> (element=w340:i32)
              n256 = Increment(x=w338) -> (x+1=w337:dbl)
              n257 = for {
                N: w340 -> [_]
                tunnel: w343 -> [w363]
                tunnel: [w361] -> w344 mode=indexing
                tunnel: [w360] -> w339 mode=indexing
                tunnel: w337 -> [_]
                i -> [w362]
                n258 = Index Array(array=w363, index (col)=w362) -> (element=w359:dbl[])  [unwired: 1 in]
                n259 = local read "Time offset"() -> (w357:i32)
                n260 = Divide(x=w357, y=10) -> (x/y=w356:dbl)
                n261 = local read "Init OP Conc"() -> (w365:dbl)
                n262 = local read "Pos Thresh"() -> (w366:dbl)
                n263 = Split 1D Array(array=w359, index=w356) -> (second subarray=w364:dbl[])  [unwired: 1 out]
                n264 = case shown="10.." w365 {
                  tunnel: w366 -> [w371 w392]
                  tunnel: [w370 w391] -> w361
                  tunnel: w364 -> [w367 w388]
                  tunnel: w356 -> [w369 w390]
                  tunnel: [w368 w389] -> w360
                  frame 10.. {
                    # "If the initial output is high, for e.g in the case of NAND, NOR, NOT"
                    n265 = for {
                      tunnel: w367 -> [w378] mode=indexing
                      tunnel: w371 -> [w375]
                      tunnel: [w377] -> w370
                      tunnel: w369 -> [w374]
                      tunnel: w367 -> [w373]
                      tunnel: [w372] -> w368
                      stop <- w376 stop-if-true
                      n266 = Less Or Equal?(x=w378, y=w375) -> (x <= y?=w379:bool)
                      n267 = case shown="True" w379 {
                        selector: w379 -> [_ w385]
                        tunnel: w378 -> [_ w387]
                        tunnel: [w380 w386] -> w377
                        tunnel: [FALSE w385] -> w376
                        tunnel: w374 -> [_ _]
                        tunnel: w373 -> [_ w384]
                        tunnel: [_ w382] -> w372
                        frame False {
                          n268 = local read "T-delay.av"() -> (w380:i32)
                        }
                        frame True {
                          n269 = Search 1D Array(1D array=w384, element=w387) -> (index of element=w382:i32)  [unwired: 1 in]
                          n270 = local read "T-Interval"() -> (w383:dbl[])
                          n271 = Index Array(array=w383, index=w382) -> (element=w386:dbl)
                        }
                      }
                    }
                  }
                  frame 0, Default {
                    # "If the initial output is low, for e.g in the case of AND,OR"
                    n272 = for {
                      tunnel: w392 -> [w397]
                      tunnel: [w399] -> w391
                      tunnel: w388 -> [w396] mode=indexing
                      tunnel: w390 -> [w395]
                      tunnel: w388 -> [w394]
                      tunnel: [w393] -> w389
                      stop <- w398 stop-if-true
                      n273 = Greater Or Equal?(x=w396, y=w397) -> (x >= y?=w400:bool)
                      n274 = case shown="True" w400 {
                        selector: w400 -> [_ w408]
                        tunnel: [w401 w405] -> w399
                        tunnel: [FALSE w408] -> w398
                        tunnel: w396 -> [_ w407]
                        tunnel: w395 -> [_ _]
                        tunnel: w394 -> [_ w406]
                        tunnel: [_ w403] -> w393
                        frame False {
                          n275 = local read "T-delay.av"() -> (w401:i32)
                        }
                        frame True {
                          n276 = Search 1D Array(1D array=w406, element=w407) -> (index of element=w403:i32)  [unwired: 1 in]
                          n277 = local read "T-Interval"() -> (w404:dbl[])
                          n278 = Index Array(array=w404, index=w403) -> (element=w405:dbl)
                        }
                      }
                    }
                  }
                }
              }
              "T-Delay" <- w344
              n279 = local read "O/p int Matrix"() -> (w336:dbl[][])
              n280 = local read "Init OP Conc"() -> (w349:dbl)
              n281 = local read "Pos Thresh"() -> (w348:dbl)
              n282 = local read "Time offset"() -> (w347:i32)
              n283 = for {
                tunnel: w336 -> [w355] mode=indexing
                tunnel: [w353] -> w333 mode=indexing
                tunnel: [w352] -> w335 mode=indexing
                tunnel: [w351] -> w334 mode=indexing
                n284 = call <vilib>:"Std Deviation and Variance.vi"("X"=w355, "Weighting (Sample)"=enum16{"Sample", "Population"}."Population") -> ("mean"=w353:dbl, "standard deviation"=w352:dbl, "variance"=w351:dbl)
              }
              n285 = Divide(x=w347, y=10) -> (x/y=w345:dbl)
              n286 = Split 1D Array(array=w333, index=w345) -> (second subarray=w350:dbl[])  [unwired: 1 out]
              n287 = case shown="0, Default" w349 {
                tunnel: w348 -> [w411 w425]
                tunnel: w350 -> [w410 w424]
                tunnel: w345 -> [w409 w423]
                tunnel: w345 -> [_ w422]
                frame 10.. {
                  # "If the initial output is high, for e.g in the case of NAND, NOR, NOT"
                  n288 = for {
                    tunnel: w410 -> [w415] mode=indexing
                    tunnel: w411 -> [w413]
                    tunnel: w409 -> [w412]
                    stop <- w414 stop-if-true
                    n289 = Less Or Equal?(x=w415, y=w413) -> (x <= y?=w416:bool)
                    n290 = case shown="True" w416 {
                      selector: w416 -> [_ w419]
                      tunnel: w415 -> [_ w420]
                      tunnel: [FALSE w419] -> w414
                      tunnel: w412 -> [_ _]
                      frame False {
                      }
                      frame True {
                        n291 = local read "OP Av"() -> (w421:dbl[])
                        n292 = Search 1D Array(1D array=w421, element=w420) -> (index of element=w418:i32)  [unwired: 1 in]
                        n293 = local write "T-Delay Idx"(w418) -> ()
                      }
                    }
                  }
                }
                frame 0, Default {
                  # "If the initial output is low, for e.g in the case of AND,OR"
                  n294 = for {
                    tunnel: w425 -> [w429]
                    tunnel: w424 -> [w428] mode=indexing
                    tunnel: w423 -> [w427]
                    tunnel: w422 -> [w426]
                    stop <- w430 stop-if-true
                    n295 = Greater Or Equal?(x=w428, y=w429) -> (x >= y?=w431:bool)
                    n296 = case shown="True" w431 {
                      selector: w431 -> [_ w436]
                      tunnel: [FALSE w436] -> w430
                      tunnel: w428 -> [_ w435]
                      tunnel: w427 -> [_ _]
                      tunnel: w426 -> [_ w434]
                      frame False {
                      }
                      frame True {
                        n297 = local read "OP Av"() -> (w437:dbl[])
                        n298 = Search 1D Array(1D array=w437, element=w435, start index (0)=w434) -> (index of element=w433:i32)
                        n299 = local write "T-Delay Idx"(w433) -> ()
                      }
                    }
                  }
                }
              }
              n300 = local write "Var"(w334) -> ()
              n301 = local write "OP Av"(w333) -> ()
              n302 = local write "SD"(w335) -> ()
              n303 = local write "TD-Idxs"(w339) -> ()
            }
            frame #1 {
              n304 = local read "T-Delay"() -> (w445:dbl[])
              n305 = for {
                tunnel: w445 -> [w466] mode=indexing
                tunnel: [w460] -> w443
                n306 = local read "Zeros"() -> (w461:dbl)
                n307 = local read "Zeros"() -> (w463:dbl)
                n308 = Increment(x=w461) -> (x+1=w462:dbl)
                n309 = Equal?(x=w466, y=0.0) -> (x = y?=w464:bool)
                n310 = Select(t=w462, s=w464, f=w463) -> (s? t:f=w460:dbl)
                n311 = local write "Zeros"(w460) -> ()
              }
              n312 = local read "Runs"() -> (w440:dbl)
              n313 = Divide(x=w440, y=2.0) -> (x/y=w438:dbl)
              n314 = Less Or Equal?(x=w443, y=w438) -> (x <= y?=w444:bool)
              n315 = case shown="True" w444 {
                tunnel: [_ w447] -> w442
                tunnel: [_ w446] -> w441
                frame False {
                }
                frame True {
                  n316 = local read "T-Delay"() -> (w450:dbl[])
                  n317 = while {
                    shift-right: [w452] -> _
                    shift-left: 0 -> [w453]
                    shift-right: [w456] -> w448
                    shift-left: w450 -> [w454]
                    stop <- w458 stop-if-true
                    n318 = Search 1D Array(1D array=w454, element=0.0, start index (0)=w453) -> (index of element=w452:i32)
                    n319 = Delete From Array(array=w454, length=1, index=w452) -> (array with subset deleted=w456:dbl[])  [unwired: 1 out]
                    n320 = Equal?(x=w452, y=-1) -> (x = y?=w458:bool)
                  }
                  "T-Delay 2" <- w448
                  n321 = call <vilib>:"Std Deviation and Variance.vi"("X"=w448, "Weighting (Sample)"=enum16{"Sample", "Population"}."Population") -> ("mean"=w447:dbl, "standard deviation"=w446:dbl)  [unwired: 1 out]
                }
              }
              "T-Delay-SD" <- w441
              n322 = local write "T-delay.av"(w442) -> ()
            }
            frame #2 {
              w484 = enum16{"Sample", "Population"}."Population" ("Weighting (Sample)")
              n323 = local read "Time offset"() -> (w479:i32)
              n324 = Divide(x=w479, y=10) -> (x/y=w477:dbl)
              n325 = local read "T-Delay Idx"() -> (w467:i32)
              n326 = local read "SD"() -> (w485:dbl[])
              n327 = local read "Var"() -> (w486:dbl[])
              n328 = local read "OP Av"() -> (w476:dbl[])
              n329 = local read "Pos Thresh"() -> (w475:dbl)
              n330 = Split 1D Array(array=w476, index=w467) -> (second subarray=w474:dbl[])  [unwired: 1 out]
              n331 = Split 1D Array(array=w485, index=w477) -> (second subarray=w483:dbl[])  [unwired: 1 out]
              n332 = Split 1D Array(array=w486, index=w477) -> (second subarray=w482:dbl[])  [unwired: 1 out]
              n333 = local read "Init OP Conc"() -> (w470:dbl)
              n334 = case shown="0, Default" w470 {
                tunnel: w475 -> [w494 w506]
                tunnel: w474 -> [w495 w505]
                tunnel: [w496 w504] -> w473
                frame 10.. {
                  # "For the case when initial output is high"
                  n335 = for {
                    tunnel: w495 -> [w503] mode=indexing
                    tunnel: w494 -> [w502]
                    tunnel: [w497] -> w496
                    n336 = local read "Var Cnt"() -> (w500:i32)
                    n337 = Greater?(x=w503, y=w502) -> (0:w498:bool)
                    n338 = local read "Var Cnt"() -> (w501:i32)
                    n339 = Increment(x=w500) -> (x+1=w499:i32)
                    n340 = Select(t=w499, s=w498, f=w501) -> (s? t:f=w497:i32)
                    n341 = local write "Var Cnt"(w497) -> ()
                  }
                }
                frame 0, Default {
                  # "For the case when initial output is low"
                  n342 = for {
                    tunnel: w505 -> [w513] mode=indexing
                    tunnel: w506 -> [w512]
                    tunnel: [w507] -> w504
                    n343 = local read "Var Cnt"() -> (w510:i32)
                    n344 = local read "Var Cnt"() -> (w511:i32)
                    n345 = Less?(x=w513, y=w512) -> (x < y?=w508:bool)
                    n346 = Increment(x=w510) -> (x+1=w509:i32)
                    n347 = Select(t=w509, s=w508, f=w511) -> (s? t:f=w507:i32)
                    n348 = local write "Var Cnt"(w507) -> ()
                  }
                }
              }
              n349 = call <vilib>:"Std Deviation and Variance.vi"("X"=w482, "Weighting (Sample)"=w484) -> ("mean"=→"Th-Var.av":dbl)  [unwired: 2 out]
              n350 = call <vilib>:"Std Deviation and Variance.vi"("X"=w483, "Weighting (Sample)"=w484) -> ("mean"=→"Th-SD.av":dbl)  [unwired: 2 out]
              n351 = local write "Zeros"(0.0 ("Zeros")) -> ()
              n352 = Array Size(array=w474) -> (size(s)=w472:i32)
              n353 = local read "T-delay.av"() -> (w469:i32)
              n354 = case shown="..-1" w469 {
                tunnel: w473 -> [_ w493]
                tunnel: w472 -> [_ w491]
                tunnel: [-1.0 w488] -> w471
                frame ..-1 {
                }
                frame 0.., Default {
                  n355 = Subtract(x=w491, y=w493) -> (x-y=w492:i32)
                  n356 = Divide(x=w492, y=w491) -> (x/y=w490:dbl)
                  n357 = Multiply(x=w490, y=100.0) -> (x*y=w488:dbl)
                }
              }
              n358 = local write "OP Consistency"(w471) -> ()
            }
          }
        }
      }
      "r2" <- w47
      "tau" <- w47
      "T" <- dbl[] [0.0] ("T")
      "L_cnt" <- w43
      "Propensities" <- w41
      "a0" <- w47
      "r1" <- w47
      "a0*r2" <- w47
      "Reac IDx" <- w43
      "Sum>a0*r2" <- FALSE ("Sum>a0*r2")
      "Reac to execute" <- w41
      "Sum of Propensities for U" <- w47
      "Nxt T" <- w47
      "Nxt Sp State (S)" <- string[] [] ("Nxt Sp State (S)")
      "Mod data" <- dbl[] [0.0, 0.0] ("Mod data")
      "Log Data Nxt" <- dbl[] [] ("Log Data Nxt")
      "Log Data matrix 2" <- dbl[][] [] ("Log Data matrix 2")
      "OP Data" <- dbl[] [] ("OP Data 2")
      "O/p Matrix" <- dbl[][] [] ("O/p Matrix")
      "Run" <- 0 ("Numeric")
      "OP Av" <- w41
      "Time array" <- dbl[] [] ("OP Data 2")
      "Time Matrix" <- dbl[][] [] ("O/p Matrix")
      "Q-Check" <- 0 ("Q-Check")
      "T-Interval" <- dbl[] [] ("OP Data 2")
      "idx" <- 0 ("Counter")
      "OP int data" <- dbl[] [] ("OP Data 2")
      "O/p int Matrix" <- dbl[][] [] ("O/p Matrix")
      "Time int Matrix" <- dbl[][] [] ("O/p Matrix")
      "Q" <- 0.0 ("Q")
      "T-delay.av" <- 0 ("index of element")
      "T-Delay Idx" <- 0 ("T-Delay Idx")
      "Var Cnt" <- 0 ("T-Delay Idx")
      "OP Consistency" <- 0.0 ("T-Delay Var")
      "SD" <- w13
      "Var" <- w13
      "TD-Idxs" <- i32[] [] ("TD-Idxs")
      "Zeros" <- 0.0 ("Zeros")
    }
    frame #2 {
      n359 = Tick Count (ms)() -> (millisecond timer value=w516:u32)
      n360 = Subtract(x=w516, y=w514) -> (x-y=→"TIME IN MS":u32)
    }
  }
